vi "校准记录.vi"(8 "error in (no error)":errorcluster, 9 "曲线模型":T1={"标液浓度1"=0.0, "测量吸光度1"=0.0, "样品1启用"=FALSE, "标液浓度2"=0.0, "测量吸光度2"=0.0, "样品2启用"=FALSE, "标液浓度3"=0.0, "测量吸光度3"=0.0, "样品3启用"=FALSE, "标液浓度4"=0.0, "测量吸光度4"=0.0, "样品4启用"=FALSE, "标液浓度5"=0.0, "测量吸光度5"=0.0, "样品5启用"=FALSE, "模型"=enum."线性", "精度"=4.0, "XY图"=[], "拟合公式"="", "r^2"=0.0, "标样一校准时间"=timestamp(0 s since 1904-01-01), "标样二校准时间"=timestamp(0 s since 1904-01-01), "标样三校准时间"=timestamp(0 s since 1904-01-01), "标样四校准时间"=timestamp(0 s since 1904-01-01), "标样五校准时间"=timestamp(0 s since 1904-01-01), "二次方程"={"c"=0.0, "x"=0.0, "x^2"=0.0}, "标定时间"=timestamp(0 s since 1904-01-01)} {"标定时间" format="%<%m/%d/%y %H:%M:%S>T"; "标样五校准时间" format="%<%m/%d/%y %H:%M:%S>T"; "标样四校准时间" format="%<%m/%d/%y %H:%M:%S>T"; "标样三校准时间" format="%<%m/%d/%y %H:%M:%S>T"; "标样二校准时间" format="%<%m/%d/%y %H:%M:%S>T"; "标样一校准时间" format="%<%m/%d/%y %H:%M:%S>T"; "r^2" format="%.7f"; "测量吸光度5" format="%#.6f"; "测量吸光度4" format="%#.6f"; "测量吸光度3" format="%#.6f"; "测量吸光度2" format="%#.6f"; "测量吸光度1" format="%#.6f"}, 10 "量程":enum16{"低量程", "高量程"}(ring), 11 "校准参数":u16(ring) items=["总氮"=2, "总磷"=1]) -> (0 "error out":errorcluster)   [LabVIEW 2016, in "斯坦道总氮V2.lvlib"]
panel:
  out "结果字符串":string
  # "校准时间"
  # "标液浓度"
  # "吸光值显示"
  # "标液一"
  # "标液二"
  # "标液三"
  # "零点"
  # "跨度"
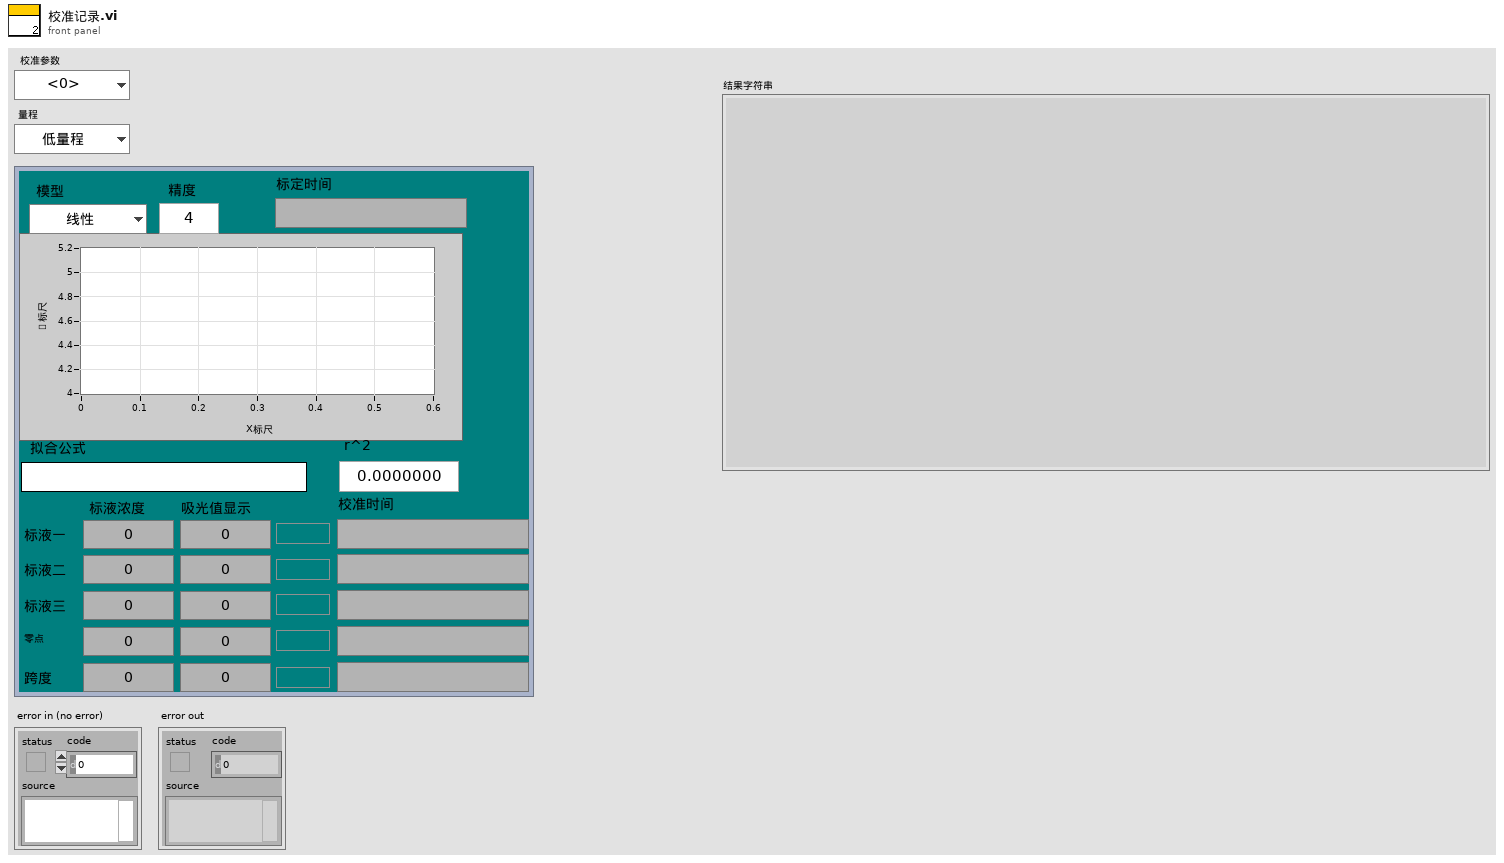
[diagram p1: front panel]
types:
  T1 = cluster{"标液浓度1":dbl, "测量吸光度1":dbl, "样品1启用":bool, "标液浓度2":dbl, "测量吸光度2":dbl, "样品2启用":bool, "标液浓度3":dbl, "测量吸光度3":dbl, "样品3启用":bool, "标液浓度4":dbl, "测量吸光度4":dbl, "样品4启用":bool, "标液浓度5":dbl, "测量吸光度5":dbl, "样品5启用":bool, "模型":enum32{"线性", "多项式"}, "精度":dbl, "XY图":cluster{"X Values":dbl[], "Y Values":dbl[]}[], "拟合公式":string, "r^2":dbl, "标样一校准时间":timestamp, "标样二校准时间":timestamp, "标样三校准时间":timestamp, "标样四校准时间":timestamp, "标样五校准时间":timestamp, "二次方程":cluster{"c":dbl, "x":dbl, "x^2":dbl}, "标定时间":timestamp}
  T2 = typedef "校准日志字段定义.ctl" = cluster{"时间":timestamp, "参数":string, "日志信息":string, "流程参数":string}
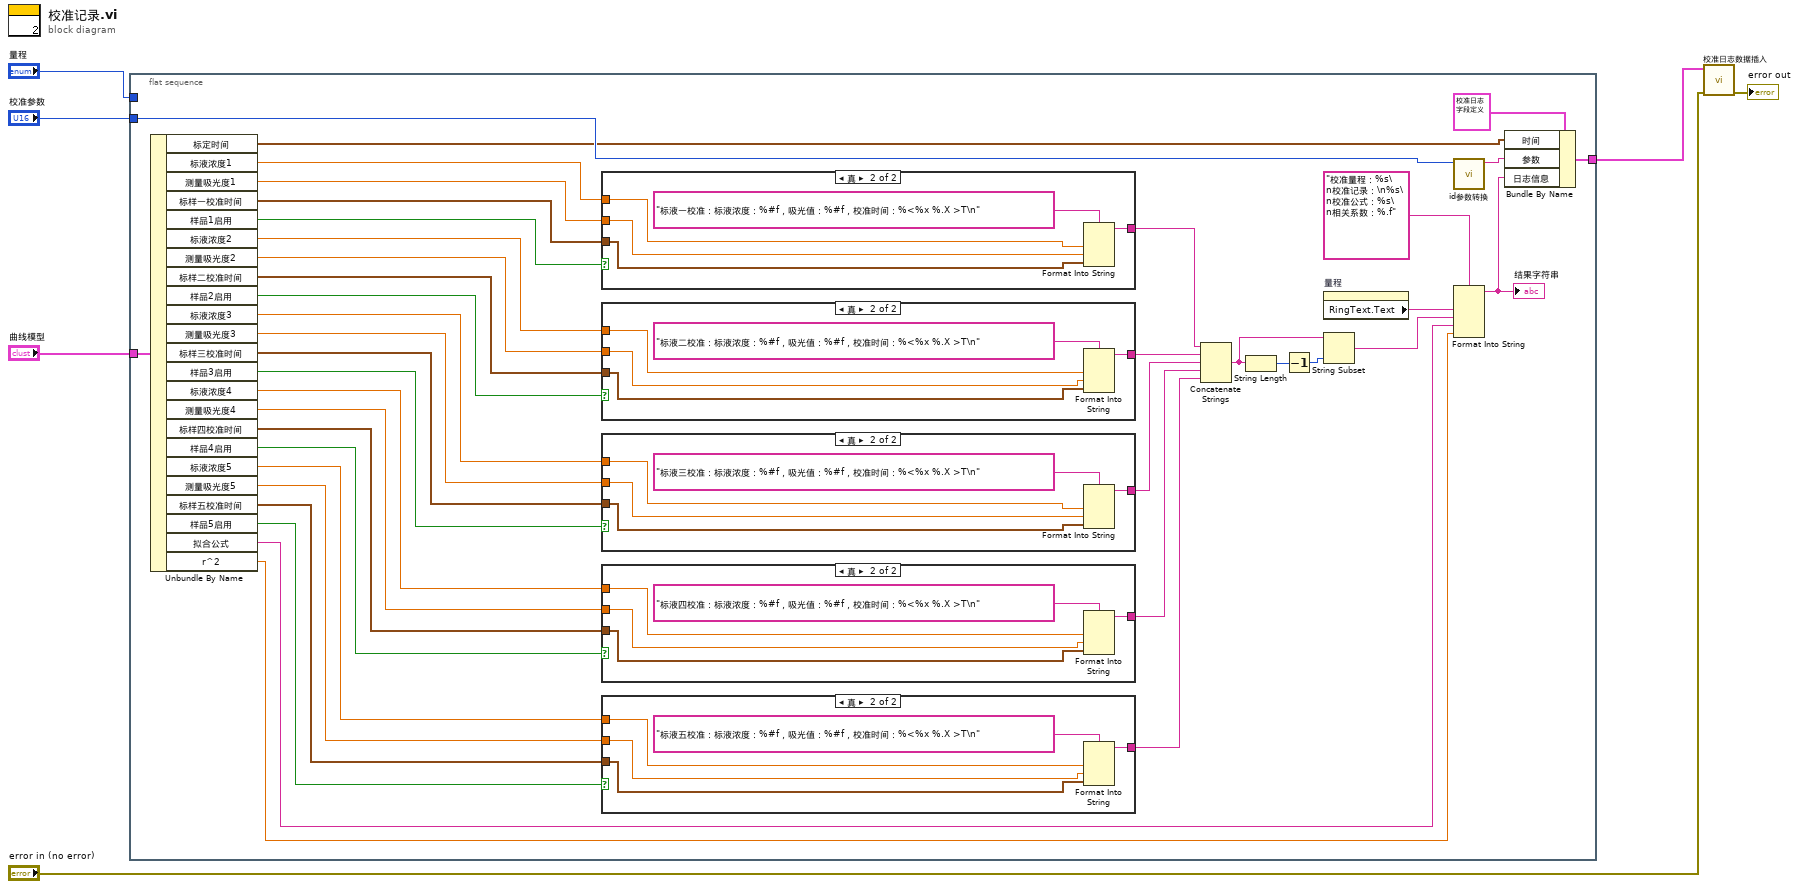
[diagram p0: block diagram]
diagram:
  n1 = flat-sequence {
    tunnel: "校准参数" -> [w46]
    tunnel: "量程" -> [_]
    tunnel: "曲线模型" -> [w41]
    tunnel: [w44] -> w3
    frame #0 {
      n2 = Unbundle By Name(w41) -> ("标定时间"=w9:timestamp, "标液浓度1"=w39:dbl, "测量吸光度1"=w38:dbl, "标样一校准时间"=w37:timestamp, "样品1启用"=w40:bool, "标液浓度2"=w36:dbl, "测量吸光度2"=w35:dbl, "标样二校准时间"=w34:timestamp, "样品2启用"=w33:bool, "标液浓度3"=w32:dbl, "测量吸光度3"=w31:dbl, "标样三校准时间"=w30:timestamp, "样品3启用"=w29:bool, "标液浓度4"=w28:dbl, "测量吸光度4"=w27:dbl, "标样四校准时间"=w26:timestamp, "样品4启用"=w25:bool, "标液浓度5"=w24:dbl, "测量吸光度5"=w23:dbl, "标样五校准时间"=w22:timestamp, "样品5启用"=w21:bool, "拟合公式"=w15:string, "r^2"=w14:dbl)
      n3 = case shown="真" w40 {
        tunnel: w39 -> [_ w70]
        tunnel: w38 -> [_ w69]
        tunnel: w37 -> [_ w68]
        tunnel: [_ w67] -> w20
        frame False {
        }
        frame True {
          n4 = Format Into String(format string="标液一校准：标液浓度：%#f，吸光值：%#f，校准时间：%<%x %.X >T\n" ("格式字符串"), w70, w69, w68) -> (resulting string=w67:string)  [unwired: 2 in, 1 out]
        }
      }
      n5 = case shown="真" w33 {
        tunnel: w36 -> [_ w65]
        tunnel: w35 -> [_ w64]
        tunnel: w34 -> [_ w63]
        tunnel: [_ w62] -> w19
        frame False {
        }
        frame True {
          n6 = Format Into String(format string="标液二校准：标液浓度：%#f，吸光值：%#f，校准时间：%<%x %.X >T\n" ("格式字符串"), w65, w64, w63) -> (resulting string=w62:string)  [unwired: 2 in, 1 out]
        }
      }
      n7 = case shown="真" w29 {
        tunnel: w32 -> [_ w60]
        tunnel: w31 -> [_ w59]
        tunnel: w30 -> [_ w58]
        tunnel: [_ w57] -> w18
        frame False {
        }
        frame True {
          n8 = Format Into String(format string="标液三校准：标液浓度：%#f，吸光值：%#f，校准时间：%<%x %.X >T\n" ("格式字符串"), w60, w59, w58) -> (resulting string=w57:string)  [unwired: 2 in, 1 out]
        }
      }
      n9 = case shown="真" w25 {
        tunnel: w28 -> [_ w55]
        tunnel: w27 -> [_ w54]
        tunnel: w26 -> [_ w53]
        tunnel: [_ w52] -> w17
        frame False {
        }
        frame True {
          n10 = Format Into String(format string="标液四校准：标液浓度：%#f，吸光值：%#f，校准时间：%<%x %.X >T\n" ("格式字符串"), w55, w54, w53) -> (resulting string=w52:string)  [unwired: 2 in, 1 out]
        }
      }
      n11 = case shown="真" w21 {
        tunnel: w24 -> [_ w50]
        tunnel: w23 -> [_ w49]
        tunnel: w22 -> [_ w48]
        tunnel: [_ w47] -> w16
        frame False {
        }
        frame True {
          n12 = Format Into String(format string="标液五校准：标液浓度：%#f，吸光值：%#f，校准时间：%<%x %.X >T\n" ("格式字符串"), w50, w49, w48) -> (resulting string=w47:string)  [unwired: 2 in, 1 out]
        }
      }
      n13 = Concatenate Strings(w20, w19, w18, w17, w16) -> (w12:string)
      n14 = String Length(string=w12) -> (length=w11:i32)
      n15 = Decrement(x=w11) -> (x-1=w10:i32)
      n16 = property on="量程" class="Enum (严格)"() -> ("RingText.Text"=w8:string)  [unwired: 2 in, 2 out]
      n17 = String Subset(string=w12, length (rest)=w10) -> (substring=w13:string)  [unwired: 1 in]
      n18 = call "id参数转换.vi"("id"=w46) -> ("table输出"=w45:string)  [unwired: 9 in, 1 out]
      n19 = Format Into String(format string="校准量程：%s\n校准记录：\n%s\n校准公式：%s\n相关系数：%.f" ("格式字符串"), w8, w13, w15, w14) -> (resulting string=w43:string)  [unwired: 2 in, 1 out]
      "结果字符串" <- w43
      n20 = Bundle By Name(cluster=T2 {"时间"=timestamp(0 s since 1904-01-01), "参数"="", "日志信息"="", "流程参数"=""} ("data"), "时间"=w9, "参数"=w45, "日志信息"=w43) -> (w44:T2)
    }
  }
  n21 = call "校准日志数据插入.vi"("data"=w3, "错误输入（无错误）"="error in (no error)") -> ("错误输出"=→"error out":errorcluster)  [unwired: 8 in]
